vi ".NET Type Builder Marshal Timebased Field.vi"(8 "error in (no error)":errorcluster, 9 ".NET Field Builder":refnum<k24>) -> (0 "error out":errorcluster, 1 ".NET Field Builder":refnum<k24>)   [LabVIEW 2018, in "TwinCAT ADS.lvclass"]
uses:
  TwinCAT ADS.lvclass
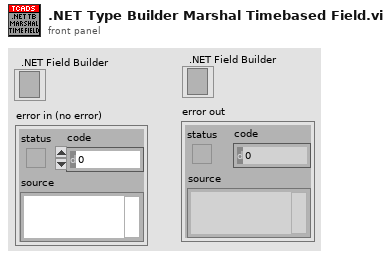
[diagram p1: front panel]
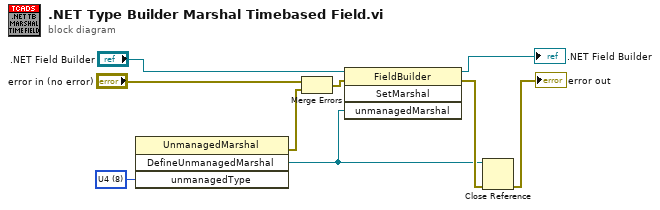
[diagram p0: block diagram]
diagram:
  w9 = 8 items=["Bool"=2, "I1"=3, "U1"=4, "I2"=5, "U2"=6, "I4"=7, "U4"=8, "I8"=9, "U8"=10, "R4"=11, "R8"=12, "Currency"=15, "BStr"=19, "LPStr"=20, "LPWStr"=21, "LPTStr"=22, "ByValTStr"=23, "IUnknown"=25, "IDispatch"=26, "Struct"=27, "Interface"=28, "SafeArray"=29, "ByValArray"=30, "SysInt"=31, "SysUInt"=32, "VBByRefStr"=34, "AnsiBStr"=35, "TBStr"=36, "VariantBool"=37, "FunctionPtr"=38, "AsAny"=40, "LPArray"=42, "LPStruct"=43, "CustomMarshaler"=44, "Error"=45, "IInspectable"=46, "HString"=47, "LPUTF8Str"=48] ("unmanagedType")
  n1 = invoke class="UnmanagedMarshal" method="DefineUnmanagedMarshal"("unmanagedType"=w9) -> (error out=w7:errorcluster, "DefineUnmanagedMarshal"=w5:refnum<k24>)  [unwired: 3 in, 2 out]
  n2 = Merge Errors("error in (no error)", w7) -> (w8:errorcluster)
  n3 = invoke class="FieldBuilder" method="SetMarshal"(reference=".NET Field Builder", error in=w8, "unmanagedMarshal"=w5) -> (reference out=→".NET Field Builder":refnum<k24>, error out=w6:errorcluster)  [unwired: 1 in, 2 out]
  n4 = Close Reference(reference=w5, error in (no error)=w6) -> (error out=→"error out":errorcluster)
